vi "Setup UI.vi"(8 "error in (no error)":errorcluster, 10 "Set UI to input? (F)":bool, 11 "PC Reader.lvclass":refnum<class "PC Reader.lvclass">) -> (0 "error out":errorcluster, 3 "PC Reader out":refnum<class "PC Reader.lvclass">)   [LabVIEW 2009, in "PC Reader.lvclass"]
doc: "Setup UI (re)constructs an object -- populates its member data -- from a front panel the user can see. The VI should be as simple as possible so that a UI loop can poll it continuously for updates. \n\nThe VI is designed to be used as a subPanel within another VI. Wire true to \"Set UI to input\" only on the first call, just after inserting this VI into a subPanel, to populate its controls with the class's current values.\n\nSetup UI is distinct from the class constructor. Class constructors are not polymorphic, yet configure dialogs need to configure objects without knowing their type -- and polymorphism is the necessary solution. Thus, Setup UI is a polymorphic class constructor. This continously polled \"Setup UI\" concept is a kludge: a better idea would be an XControl, but those require a steeper learning curve."
uses:
  PC Reader.lvclass
  PC Reader.lvclass/PC Reader.ctl
panel:
  in  "Gate B Ref":enum16{"t=0", "t=T/4", "t=T/2", "t=3T/4"}(ring)
  in  "Gate A Ref":enum16{"t=0", "t=T/4", "t=T/2", "t=3T/4"}(ring)
  out "Gate B Delay Actual":dbl[unit]
  out "Gate A Delay Actual":dbl[unit]
  in  "start vs mid. of gate":bool caption="Delays measured to"
  in  "Gate B %":dbl
  in  "Gate A %":dbl
  in  "time vs percent":bool caption="Width in"
  out "Gate B Mode":enum16{"CW", "Fixed", "Scan"}(ring)
  out "Gate A Mode":enum16{"CW", "Fixed", "Scan"}(ring)
  in  "Gate B Width":dbl[unit]
  in  "Gate B Delay":dbl[unit]
  in  "Gate A Delay":dbl[unit]
  in  "Gate A Width":dbl[unit]
  in  "Ext. Trigger?":bool
  in  "Ext. Trig. Freq.":dbl[unit]
  in  "Count Time":dbl[unit] format="%#_4g"
  in  "Send first pt to PC":bool
  in  "indAw?":bool
  in  "indAd?":bool
  in  "indBw?":bool
  in  "indBd?":bool
  # "Photon Counter Setup"
  # "Track ind.var.?\n(assumes in ns)"
  # "(PEM = 42.0762 kHz)"
  # "(If tracking, these times represent \nthe values for the first pt.)"
  # "PURE VIRTUAL\nMETHOD CALLED!"
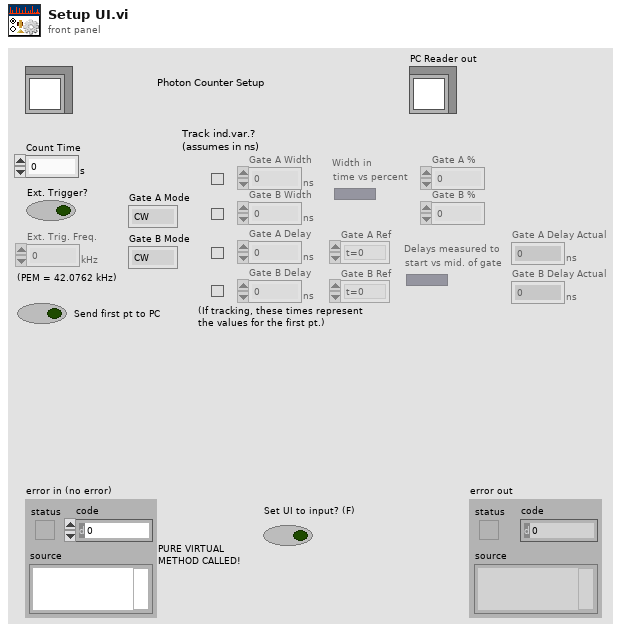
[diagram p1: front panel]
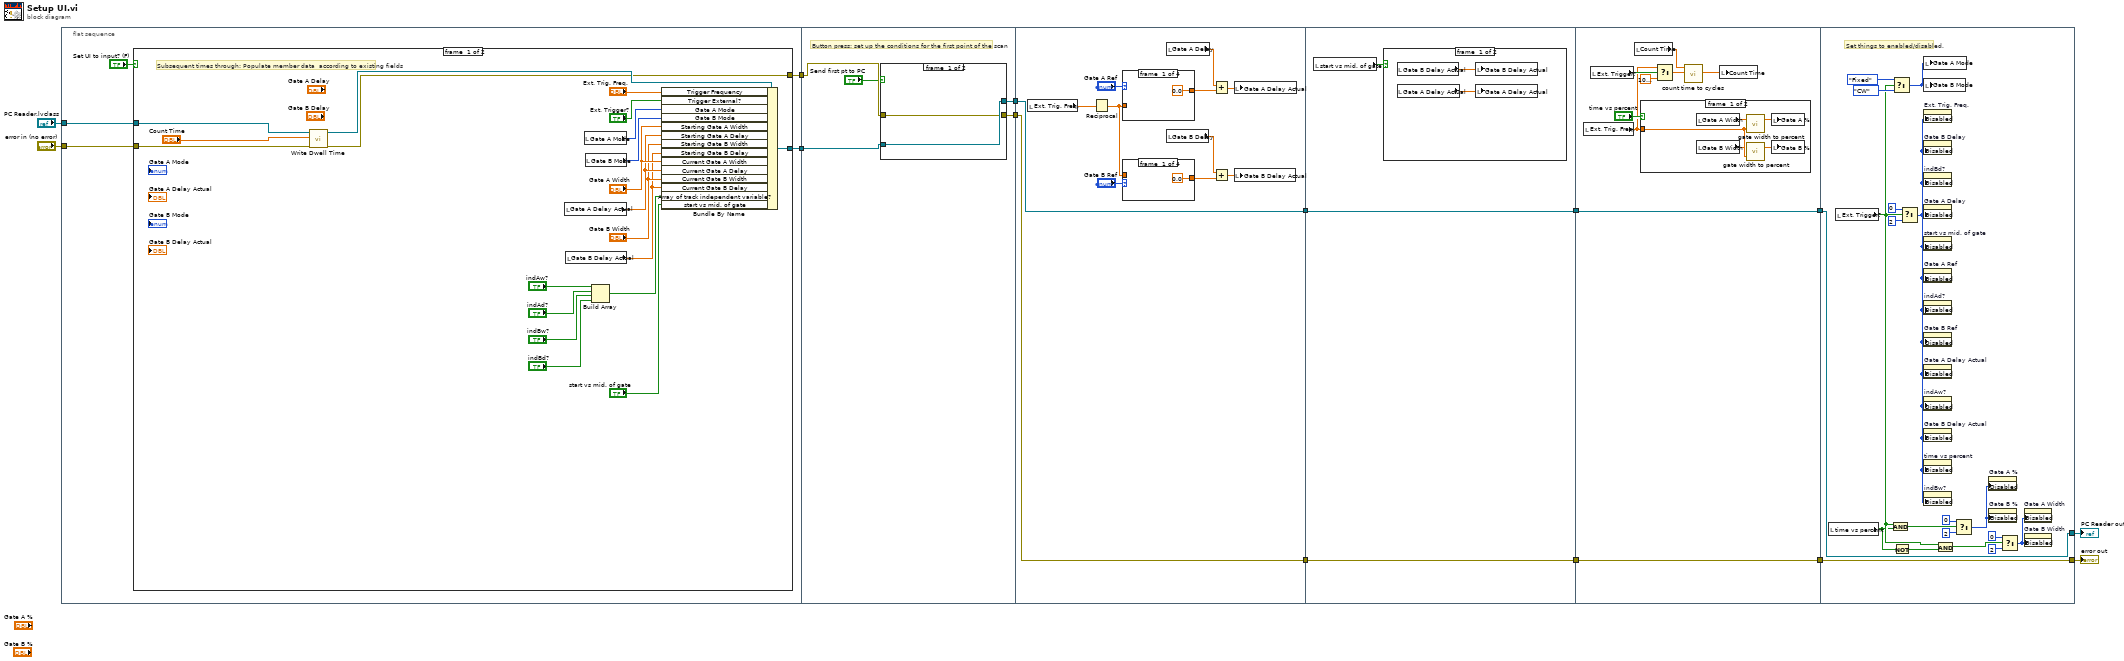
[diagram p0: block diagram]
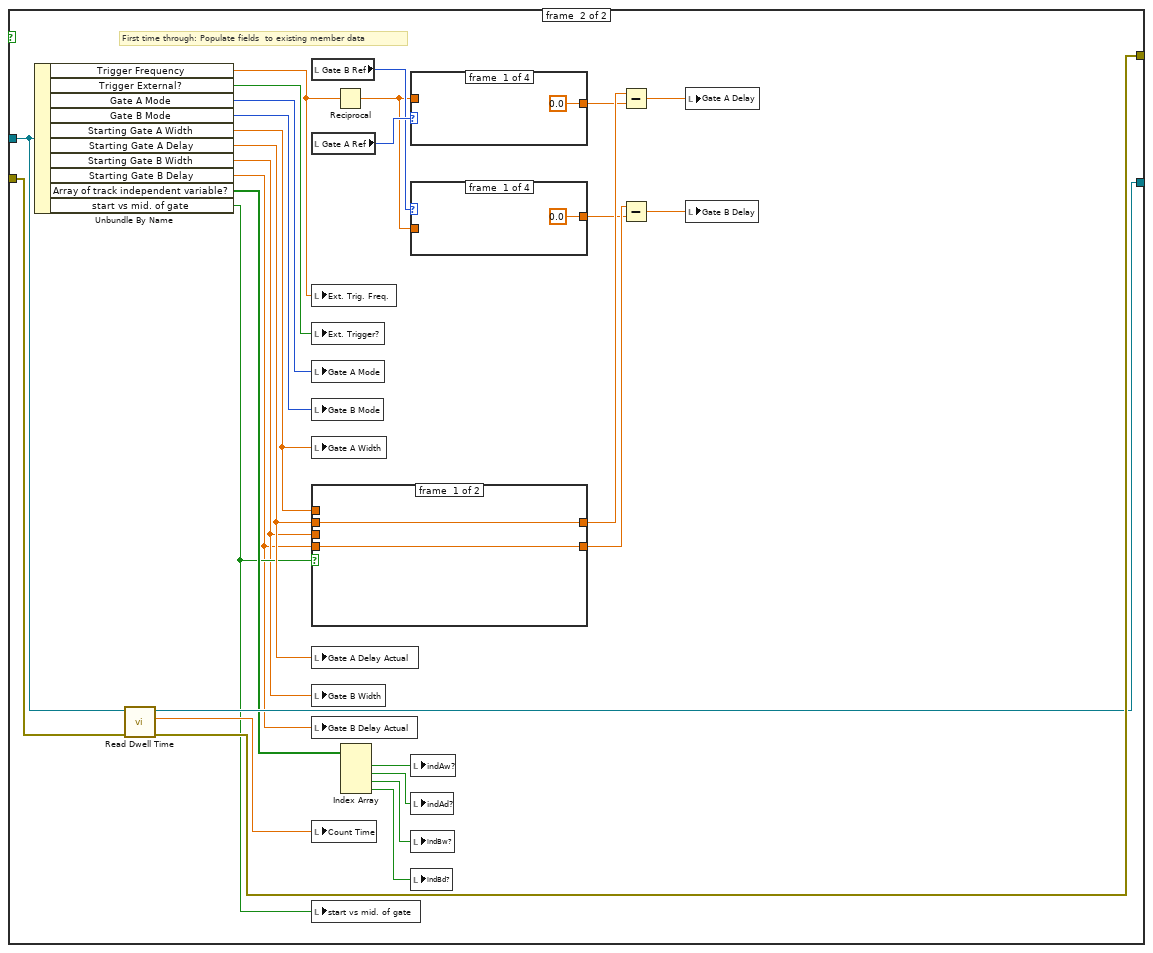
[diagram p2: hidden frame]
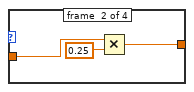
[diagram p3: hidden frame]
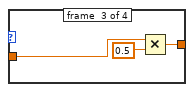
[diagram p4: hidden frame]
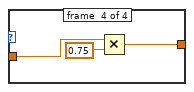
[diagram p5: hidden frame]
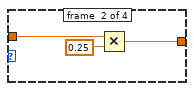
[diagram p6: hidden frame]
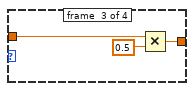
[diagram p7: hidden frame]
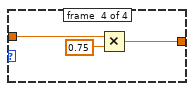
[diagram p8: hidden frame]
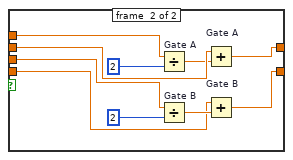
[diagram p9: hidden frame]
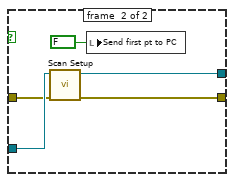
[diagram p10: hidden frame]
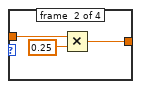
[diagram p11: hidden frame]
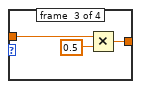
[diagram p12: hidden frame]
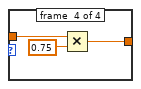
[diagram p13: hidden frame]
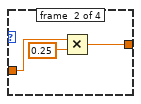
[diagram p14: hidden frame]
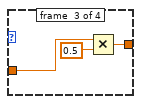
[diagram p15: hidden frame]
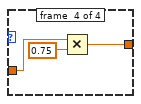
[diagram p16: hidden frame]
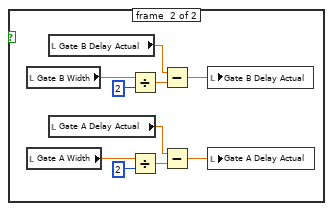
[diagram p17: hidden frame]
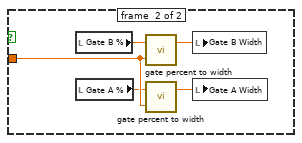
[diagram p18: hidden frame]
diagram:
  n1 = flat-sequence {
    tunnel: "error in (no error)" -> [w16]
    tunnel: [w19] -> w2
    tunnel: [w15] -> w1
    tunnel: "PC Reader.lvclass" -> [w17]
    tunnel: w2 -> [w104]
    tunnel: w1 -> [w103]
    tunnel: [w102] -> w8
    tunnel: [w100] -> w6
    tunnel: w8 -> [w123]
    tunnel: [w123] -> w7
    tunnel: w6 -> [w122]
    tunnel: [w122] -> w5
    tunnel: w7 -> [w146]
    tunnel: [w146] -> w10
    tunnel: w5 -> [w145]
    tunnel: [w145] -> w9
    tunnel: w10 -> [w167]
    tunnel: [w167] -> w12
    tunnel: w9 -> [w166]
    tunnel: [w166] -> w11
    tunnel: w12 -> [w196]
    tunnel: [w195] -> w3
    tunnel: [w196] -> w13
    tunnel: w11 -> [w195]
    frame #0 {
      n2 = case shown="True" "Set UI to input? (F)" {
        tunnel: [w31 w58] -> w19
        tunnel: w17 -> [w32 w59]
        tunnel: [w28 w60] -> w15
        tunnel: w16 -> [w27 w61]
        frame #0 {
          # "Subsequent times through: Populate member data  according to existing fields"
          n3 = call-dynamic "Write Dwell Time.vi"("error in (no error)"=w27, "Dwell Time"="Count Time", "Reader.lvclass in"=w32) -> ("error out"=w28:errorcluster, "Reader.lvclass out"=w30:refnum<class "PC Reader.lvclass">)  [unwired: 7 out]
          n4 = local read "Gate A Delay Actual"() -> (w24:dbl[unit])
          n5 = local read "Gate B Delay Actual"() -> (w22:dbl[unit])
          n6 = local read "Gate A Mode"() -> (w33:enum16{"CW", "Fixed", "Scan"})
          n7 = local read "Gate B Mode"() -> (w26:enum16{"CW", "Fixed", "Scan"})
          n8 = Build Array("indAw?", "indAd?", "indBw?", "indBd?") -> (w21:bool[])
          n9 = Bundle By Name(cluster=w30, "Trigger Frequency"="Ext. Trig. Freq.", "Trigger External?"="Ext. Trigger?", "Gate A Mode"=w33, "Gate B Mode"=w26, "Starting Gate A Width"="Gate A Width", "Starting Gate A Delay"=w24, "Starting Gate B Width"="Gate B Width", "Starting Gate B Delay"=w22, "Current Gate A Width"="Gate A Width", "Current Gate A Delay"=w24, "Current Gate B Width"="Gate B Width", "Current Gate B Delay"=w22, "Array of track independent variable?"=w21, "start vs mid. of gate"="start vs mid. of gate") -> (w31:refnum<class "PC Reader.lvclass">)
        }
        frame #1 {
          # "First time through: Populate fields  to existing member data"
          n10 = Unbundle By Name(w59) -> ("Trigger Frequency"=w54:dbl[unit], "Trigger External?"=w63:bool, "Gate A Mode"=w62:u16, "Gate B Mode"=w48:u16, "Starting Gate A Width"=w46:dbl[unit], "Starting Gate A Delay"=w47:dbl[unit], "Starting Gate B Width"=w43:dbl[unit], "Starting Gate B Delay"=w42:dbl[unit], "Array of track independent variable?"=w45:bool[], "start vs mid. of gate"=w44:bool)
          n11 = call-dynamic "Read Dwell Time.vi"("error in (no error)"=w61, "Reader.lvclass in"=w59) -> ("error out"=w60:errorcluster, "Dwell Time"=w57:dbl[unit], "Reader.lvclass out"=w58:refnum<class "PC Reader.lvclass">)  [unwired: 7 out]
          n12 = local read "Gate B Ref"() -> (w55:enum16{"t=0", "t=T/4", "t=T/2", "t=3T/4"})
          n13 = local read "Gate A Ref"() -> (w56:enum16{"t=0", "t=T/4", "t=T/2", "t=3T/4"})
          n14 = local write "Ext. Trig. Freq."(w54) -> ()
          n15 = local write "Ext. Trigger?"(w63) -> ()
          n16 = local write "Gate A Mode"(w62) -> ()
          n17 = local write "Gate B Mode"(w48) -> ()
          n18 = local write "Gate A Width"(w46) -> ()
          n19 = case shown="False" w44 {
            tunnel: [w89 w93] -> w52
            tunnel: w47 -> [w89 w97]
            tunnel: [w88 w92] -> w49
            tunnel: w46 -> [_ w94]
            tunnel: w43 -> [_ w91]
            tunnel: w42 -> [w88 w90]
            frame #0 {
            }
            frame #1 {
              n20 = Divide "Gate A"(x=w94, y=2) -> (x/y=w96:dbl[unit])
              n21 = Divide "Gate B"(x=w91, y=2) -> (x/y=w95:dbl[unit])
              n22 = Add "Gate A"(x=w97, y=w96) -> (x+y=w93:dbl[unit])
              n23 = Add "Gate B"(x=w90, y=w95) -> (x+y=w92:dbl[unit])
            }
          }
          n24 = local write "Gate A Delay Actual"(w47) -> ()
          n25 = local write "Gate B Width"(w43) -> ()
          n26 = local write "Gate B Delay Actual"(w42) -> ()
          n27 = local write "Count Time"(w57) -> ()
          n28 = local write "start vs mid. of gate"(w44) -> ()
          n29 = Reciprocal(x=w54) -> (1/x=w53:dbl[unit])
          n30 = Index Array(array=w45) -> (element #1=w64:bool, element #2=w65:bool, element #3=w66:bool, element #4=w67:bool)  [unwired: 4 in]
          n31 = case shown="\"t=T/4\"" w56 {
            tunnel: [dbl[unit] 0.0 ("x/y") w79 w82 w85] -> w51
            tunnel: w53 -> [_ w80 w83 w86]
            frame #0 {
            }
            frame #1 {
              n32 = Multiply(x=w80, y=0.25) -> (x*y=w79:dbl[unit])
            }
            frame #2 {
              n33 = Multiply(x=w83, y=0.5) -> (x*y=w82:dbl[unit])
            }
            frame #3 {
              n34 = Multiply(x=w86, y=0.75) -> (x*y=w85:dbl[unit])
            }
          }
          n35 = case shown="\"t=3T/4\"" w55 {
            tunnel: [dbl[unit] 0.0 ("x/y") w69 w72 w75] -> w40
            tunnel: w53 -> [_ w70 w73 w76]
            frame #0 {
            }
            frame #1 {
              n36 = Multiply(x=w70, y=0.25) -> (x*y=w69:dbl[unit])
            }
            frame #2 {
              n37 = Multiply(x=w73, y=0.5) -> (x*y=w72:dbl[unit])
            }
            frame #3 {
              n38 = Multiply(x=w76, y=0.75) -> (x*y=w75:dbl[unit])
            }
          }
          n39 = local write "indAw?"(w64) -> ()
          n40 = local write "indAd?"(w65) -> ()
          n41 = local write "indBw?"(w66) -> ()
          n42 = local write "indBd?"(w67) -> ()
          n43 = Subtract(x=w52, y=w51) -> (x-y=w50:dbl[unit])
          n44 = Subtract(x=w49, y=w40) -> (x-y=w41:dbl[unit])
          n45 = local write "Gate A Delay"(w50) -> ()
          n46 = local write "Gate B Delay"(w41) -> ()
        }
      }
    }
    frame #1 {
      # "Button press: set up the conditions for the first point of the scan"
      n47 = case shown="True" "Send first pt to PC" {
        tunnel: [w106 w107] -> w100
        tunnel: [w105 w108] -> w102
        tunnel: w104 -> [w106 w110]
        tunnel: w103 -> [w105 w109]
        frame #0 {
        }
        frame #1 {
          n48 = call-dynamic "Scan Setup.vi"("error in (no error)"=w109, "PC Reader in"=w110) -> ("error out"=w108:errorcluster, "PC Reader out"=w107:refnum<class "PC Reader.lvclass">)  [unwired: 8 out]
          n49 = local write "Send first pt to PC"(FALSE ("Send conds for first point to PG")) -> ()
        }
      }
    }
    frame #2 {
      n50 = local read "Ext. Trig. Freq."() -> (w119:dbl[unit])
      n51 = Reciprocal(x=w119) -> (1/x=w118:dbl[unit])
      n52 = case shown="\"t=0\", Default" "Gate A Ref" {
        tunnel: w118 -> [_ w136 w139 w142]
        tunnel: [dbl[unit] 0.0 ("x/y") w135 w138 w141] -> w116
        frame #0 {
        }
        frame #1 {
          n53 = Multiply(x=w136, y=0.25) -> (x*y=w135:dbl[unit])
        }
        frame #2 {
          n54 = Multiply(x=w139, y=0.5) -> (x*y=w138:dbl[unit])
        }
        frame #3 {
          n55 = Multiply(x=w142, y=0.75) -> (x*y=w141:dbl[unit])
        }
      }
      n56 = case shown="\"t=T/4\"" "Gate B Ref" {
        tunnel: w118 -> [_ w126 w129 w132]
        tunnel: [dbl[unit] 0.0 ("x/y") w125 w128 w131] -> w113
        frame #0 {
        }
        frame #1 {
          n57 = Multiply(x=w126, y=0.25) -> (x*y=w125:dbl[unit])
        }
        frame #2 {
          n58 = Multiply(x=w129, y=0.5) -> (x*y=w128:dbl[unit])
        }
        frame #3 {
          n59 = Multiply(x=w132, y=0.75) -> (x*y=w131:dbl[unit])
        }
      }
      n60 = local read "Gate A Delay"() -> (w117:dbl[unit])
      n61 = local read "Gate B Delay"() -> (w114:dbl[unit])
      n62 = Add(x=w117, y=w116) -> (x+y=w115:dbl[unit])
      n63 = Add(x=w114, y=w113) -> (x+y=w112:dbl[unit])
      n64 = local write "Gate A Delay Actual"(w115) -> ()
      n65 = local write "Gate B Delay Actual"(w112) -> ()
    }
    frame #3 {
      n66 = local read "start vs mid. of gate"() -> (w144:bool)
      n67 = case shown="True" w144 {
        frame #0 {
          n68 = local read "Gate B Delay Actual"() -> (w147:dbl[unit])
          n69 = local read "Gate A Delay Actual"() -> (w148:dbl[unit])
          n70 = local write "Gate B Delay Actual"(w147) -> ()
          n71 = local write "Gate A Delay Actual"(w148) -> ()
        }
        frame #1 {
          n72 = local read "Gate B Width"() -> (w151:dbl[unit])
          n73 = local read "Gate A Width"() -> (w155:dbl[unit])
          n74 = local read "Gate B Delay Actual"() -> (w152:dbl[unit])
          n75 = local read "Gate A Delay Actual"() -> (w156:dbl[unit])
          n76 = Divide(x=w151, y=2) -> (x/y=w153:dbl[unit])
          n77 = Divide(x=w155, y=2) -> (x/y=w154:dbl[unit])
          n78 = Subtract(x=w152, y=w153) -> (x-y=w149:dbl[unit])
          n79 = Subtract(x=w156, y=w154) -> (x-y=w150:dbl[unit])
          n80 = local write "Gate B Delay Actual"(w149) -> ()
          n81 = local write "Gate A Delay Actual"(w150) -> ()
        }
      }
    }
    frame #4 {
      n82 = local read "Ext. Trig. Freq."() -> (w162:dbl[unit])
      n83 = local read "Ext. Trigger?"() -> (w163:bool)
      n84 = local read "Count Time"() -> (w164:dbl[unit])
      n85 = case shown="True" "time vs percent" {
        tunnel: w162 -> [w172 w175]
        frame #0 {
          n86 = local read "Gate A Width"() -> (w171:dbl[unit])
          n87 = local read "Gate B Width"() -> (w170:dbl[unit])
          n88 = call "gate width to percent.vi"("Trigger Freq"=w172, "Gate width"=w171) -> ("Gate %"=w169:dbl)  [unwired: 1 out]
          n89 = call "gate width to percent.vi"("Trigger Freq"=w172, "Gate width"=w170) -> ("Gate %"=w168:dbl)  [unwired: 1 out]
          n90 = local write "Gate A %"(w169) -> ()
          n91 = local write "Gate B %"(w168) -> ()
        }
        frame #1 {
          n92 = local read "Gate B %"() -> (w173:dbl)
          n93 = local read "Gate A %"() -> (w174:dbl)
          n94 = call "gate percent to width.vi"("Trigger Freq"=w175, "Gate %"=w173) -> ("Gate width"=w177:dbl[unit])  [unwired: 1 out]
          n95 = call "gate percent to width.vi"("Trigger Freq"=w175, "Gate %"=w174) -> ("Gate width"=w176:dbl[unit])  [unwired: 1 out]
          n96 = local write "Gate B Width"(w177) -> ()
          n97 = local write "Gate A Width"(w176) -> ()
        }
      }
      n98 = Select(t=w162, s=w163, f=dbl[unit] 10000000.0 ("Trigger Freq")) -> (s? t:f=w160:dbl[unit])
      n99 = call "count time to cycles.vi"("Trigger Freq"=w160, "Count Time Set"=w164) -> ("Count Time Current"=w159:dbl[unit])  [unwired: 1 in, 4 out]
      n100 = local write "Count Time"(w159) -> ()
    }
    frame #5 {
      # "Set things to enabled/disabled."
      n101 = local read "time vs percent"() -> (w179:bool)
      n102 = local read "Ext. Trigger?"() -> (w180:bool)
      n103 = And(x=w180, y=w179) -> (x .and. y?=w187:bool)
      n104 = Select(t=enum16{"CW", "Fixed", "Scan"}."Fixed" ("Gate A Mode"), s=w180, f=enum16{"CW", "Fixed", "Scan"}."CW" ("Gate A Mode")) -> (s? t:f=w192:enum16{"CW", "Fixed", "Scan"})
      n105 = Not(x=w179) -> (.not. x?=w181:bool)
      n106 = Select(t=0, s=w180, f=2) -> (s? t:f=w178:i32)
      n107 = local write "Gate A Mode"(w192) -> ()
      n108 = local write "Gate B Mode"(w192) -> ()
      n109 = property on="Ext. Trig. Freq." class="DigNum (strict)"("Disabled"=w178) -> ()  [unwired: 2 in, 2 out]
      n110 = property on="Gate B Delay" class="DigNum (strict)"("Disabled"=w178) -> ()  [unwired: 2 in, 2 out]
      n111 = property on="indBd?" class="Bool (strict)"("Disabled"=w178) -> ()  [unwired: 2 in, 2 out]
      n112 = property on="Gate A Delay" class="DigNum (strict)"("Disabled"=w178) -> ()  [unwired: 2 in, 2 out]
      n113 = property on="start vs mid. of gate" class="Bool (strict)"("Disabled"=w178) -> ()  [unwired: 2 in, 2 out]
      n114 = property on="Gate A Ref" class="Enum (strict)"("Disabled"=w178) -> ()  [unwired: 2 in, 2 out]
      n115 = property on="indAd?" class="Bool (strict)"("Disabled"=w178) -> ()  [unwired: 2 in, 2 out]
      n116 = property on="Gate B Ref" class="Enum (strict)"("Disabled"=w178) -> ()  [unwired: 2 in, 2 out]
      n117 = property on="Gate A Delay Actual" class="DigNum (strict)"("Disabled"=w178) -> ()  [unwired: 2 in, 2 out]
      n118 = property on="indAw?" class="Bool (strict)"("Disabled"=w178) -> ()  [unwired: 2 in, 2 out]
      n119 = property on="Gate B Delay Actual" class="DigNum (strict)"("Disabled"=w178) -> ()  [unwired: 2 in, 2 out]
      n120 = property on="time vs percent" class="Bool (strict)"("Disabled"=w178) -> ()  [unwired: 2 in, 2 out]
      n121 = property on="indBw?" class="Bool (strict)"("Disabled"=w178) -> ()  [unwired: 2 in, 2 out]
      n122 = And(x=w180, y=w181) -> (x .and. y?=w183:bool)
      n123 = Select(t=0, s=w187, f=2) -> (s? t:f=w186:i32)
      n124 = property on="Gate A %" class="DigNum (strict)"("Disabled"=w186) -> ()  [unwired: 2 in, 2 out]
      n125 = property on="Gate B %" class="DigNum (strict)"("Disabled"=w186) -> ()  [unwired: 2 in, 2 out]
      n126 = Select(t=0, s=w183, f=2) -> (s? t:f=w182:i32)
      n127 = property on="Gate A Width" class="DigNum (strict)"("Disabled"=w182) -> ()  [unwired: 2 in, 2 out]
      n128 = property on="Gate B Width" class="DigNum (strict)"("Disabled"=w182) -> ()  [unwired: 2 in, 2 out]
    }
  }
  "error out" <- w13
  "PC Reader out" <- w3
